vi "SubVI2.vi"(8 "y":dbl, 9 "x":dbl) -> (0 "x+y":dbl)   [LabVIEW 2022 SP3]
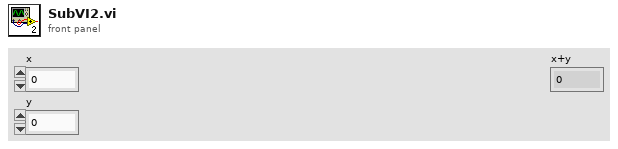
[diagram p1: front panel]
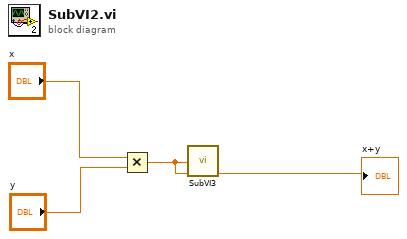
[diagram p0: block diagram]
diagram:
  n1 = Multiply(x="x", y="y") -> (x*y=w2:dbl)
  n2 = call "SubVI3.vi"("x"=w2, "y"=w2) -> ("x+y"=→"x+y":dbl)  [unwired: 7 in]
